vi "joystick.vi"() -> ()   [LabVIEW 2014]
panel:
  in  "USB settings":cluster{"S/N":string, "USB Search?":bool}={"S/N"="", "USB Search?"=TRUE}
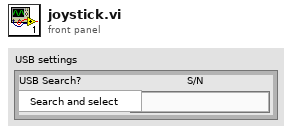
[diagram p1: front panel]
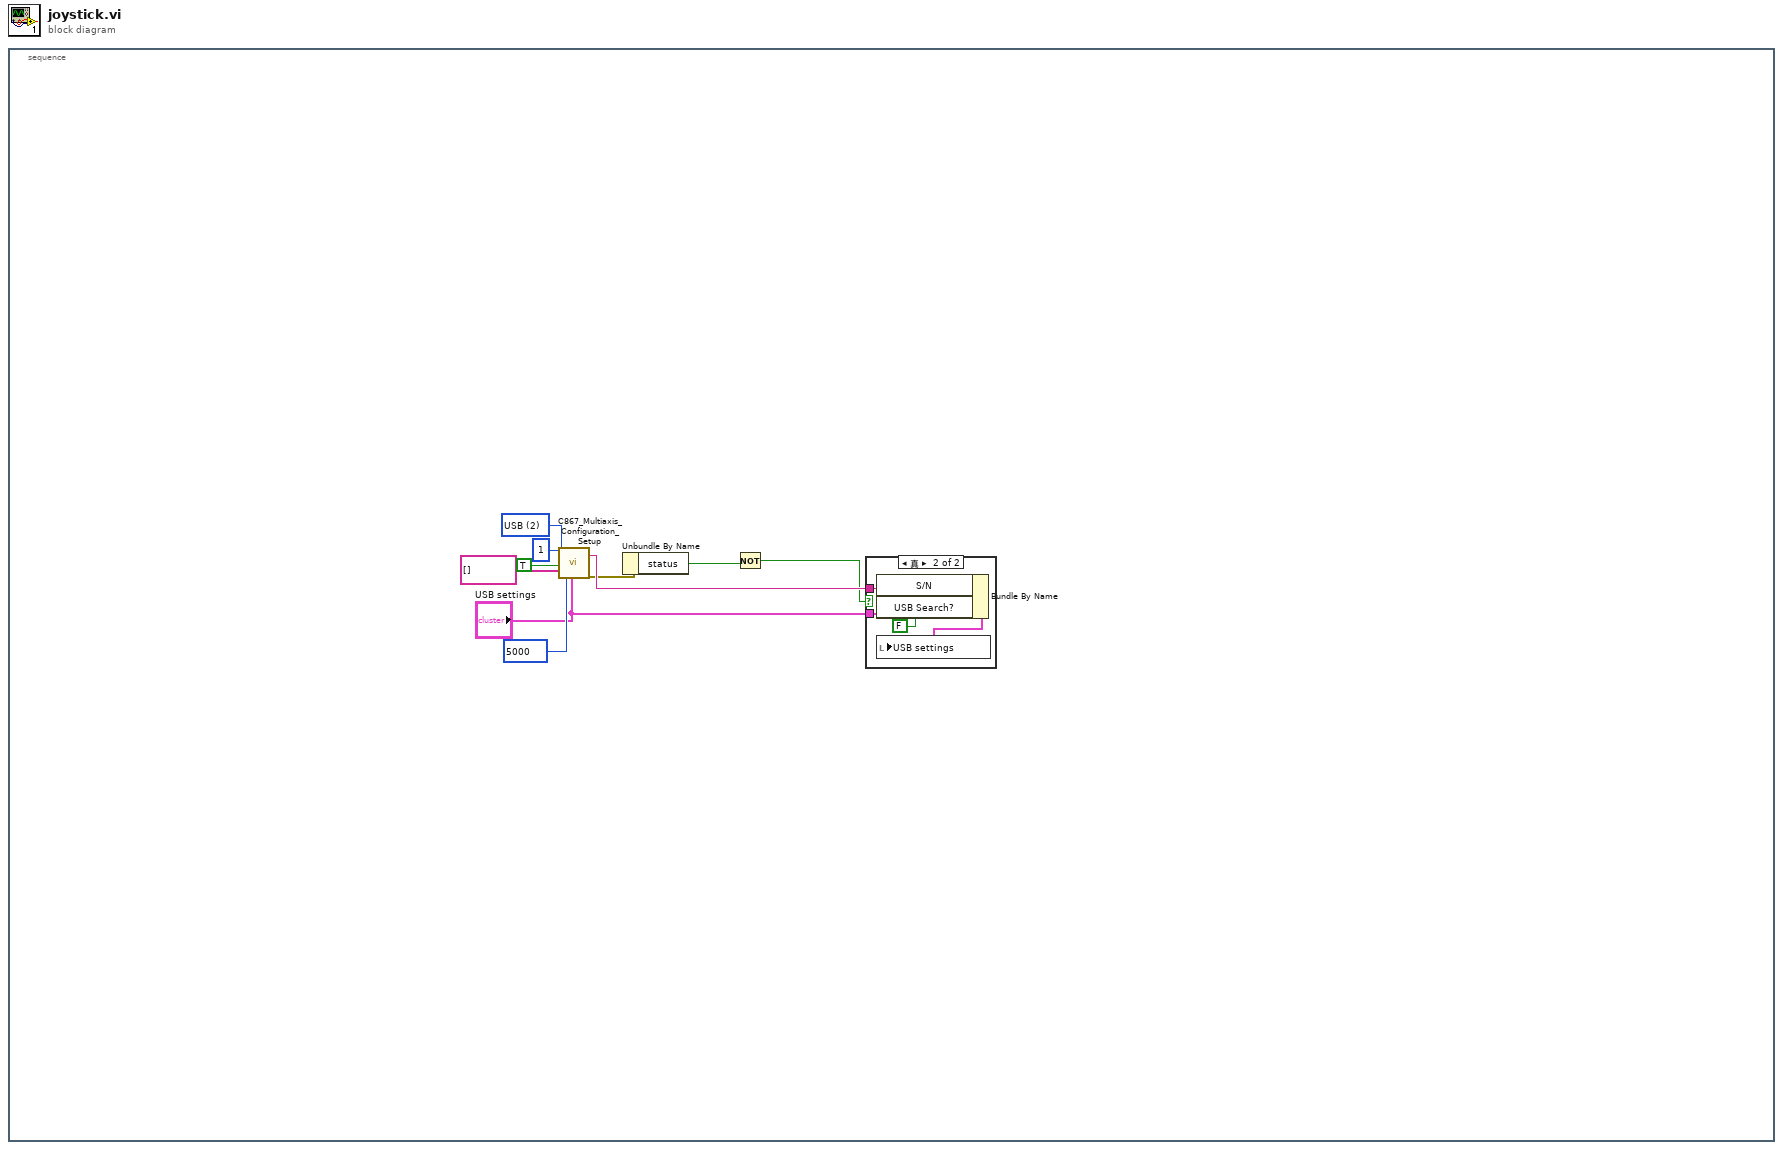
[diagram p0: block diagram]
diagram:
  n1 = stacked-sequence {
    frame #0 {
      w9 = u16 2 items=["RS232", "RS232 DaisyChain", "USB"] ("Interface")
      n2 = call "C867_Multiaxis_Configuration_Setup.vi"("System no."=1, "Interface"=w9, "All axes?"=TRUE, "Axes to move"=string[] [], "Timeout"=u32 5000, "USB settings"="USB settings") -> ("SN out"=w5:string, "error out"=w4:errorcluster)  [unwired: 7 in, 5 out]
      n3 = Unbundle By Name(w4) -> ("status"=w3:bool)
      n4 = Not(x=w3) -> (.not. x?=w2:bool)
      n5 = case shown="真" w2 {
        tunnel: "USB settings" -> [_ w14]
        tunnel: w5 -> [_ w13]
        frame False {
        }
        frame True {
          n6 = Bundle By Name(cluster=w14, "S/N"=w13, "USB Search?"=FALSE) -> (w11:cluster{"S/N":string, "USB Search?":bool})
          n7 = local write "USB settings"(w11) -> ()
        }
      }
    }
  }
